vi "allStatus.vi"(4 "intake":bool, 6 "drive":bool, 8 "gear":bool, 9 "shooter":bool, 10 "hopper1":bool, 11 "hopper0":bool) -> ()   [LabVIEW 2016]
uses:
  2ndContollerStatus.vi
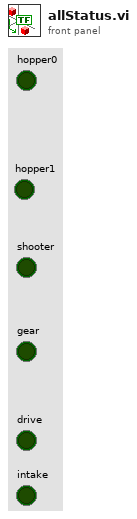
[diagram p1: front panel]
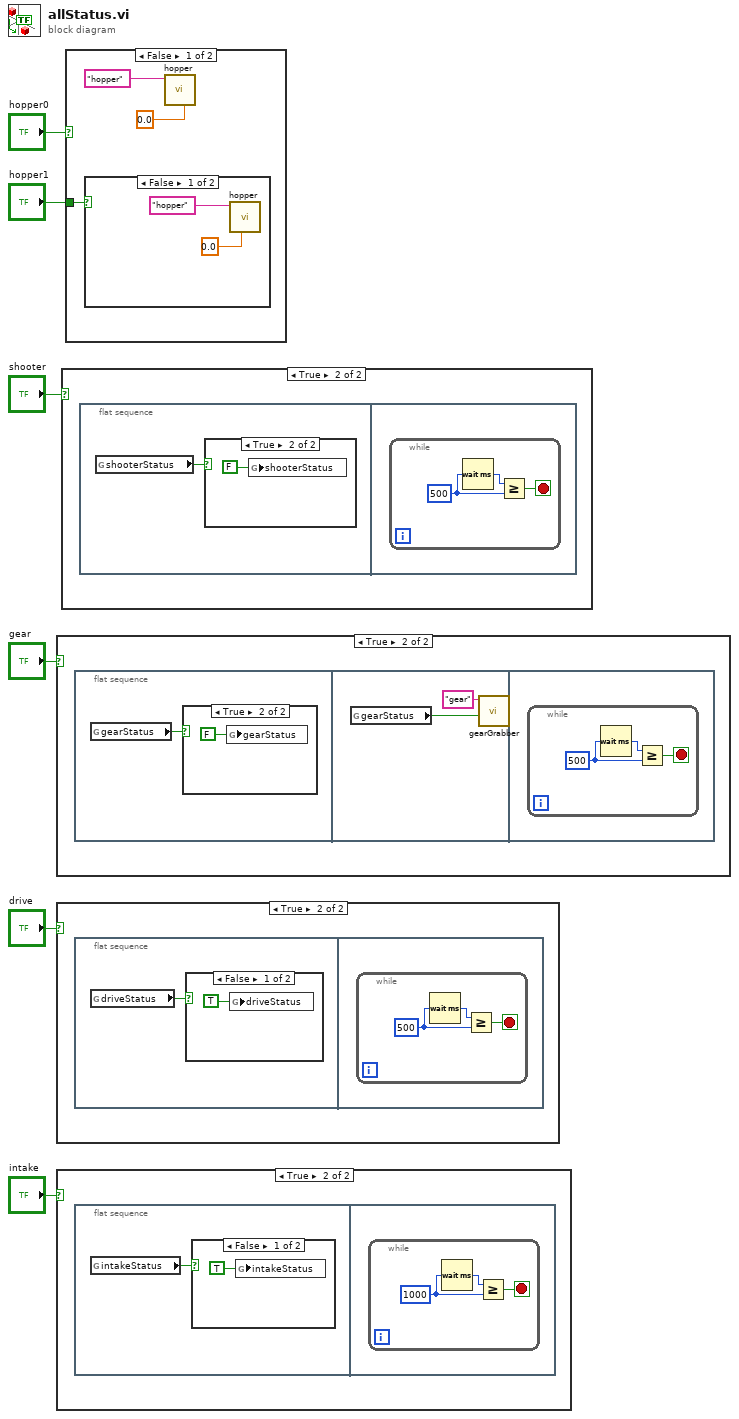
[diagram p0: block diagram]
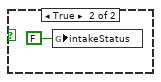
[diagram p3: hidden frame]
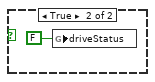
[diagram p5: hidden frame]
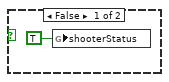
[diagram p7: hidden frame]
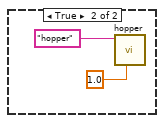
[diagram p8: hidden frame]
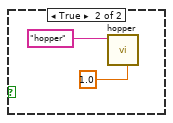
[diagram p9: hidden frame]
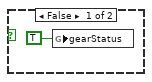
[diagram p11: hidden frame]
diagram:
  n1 = case shown="True" "gear" {
    frame False {
    }
    frame True {
      n2 = flat-sequence {
        frame #0 {
          n3 = global read "2ndContollerStatus.vi" "gearStatus"() -> (w7:bool)
          n4 = case shown="True" w7 {
            frame False {
              n5 = global write "2ndContollerStatus.vi" "gearStatus"(TRUE ("gearStatus")) -> ()
            }
            frame True {
              n6 = global write "2ndContollerStatus.vi" "gearStatus"(FALSE ("gearStatus")) -> ()
            }
          }
        }
        frame #1 {
          n7 = global read "2ndContollerStatus.vi" "gearStatus"() -> (w10:bool)
          n8 = call "gearGrabber.vi"("gearStatus"=w10, "gear"="gear") -> ()  [unwired: 9 in, 1 out]
        }
        frame #2 {
          n9 = while {
            stop <- w14 stop-if-true
            w12 = u32 500 ("milliseconds to wait")
            n10 = Wait (ms)(milliseconds to wait=w12) -> (millisecond timer value=w13:u32)
            n11 = Greater Or Equal?(x=w13, y=w12) -> (x >= y?=w14:bool)
          }
        }
      }
    }
  }
  n12 = case shown="True" "drive" {
    frame False {
    }
    frame True {
      n13 = flat-sequence {
        frame #0 {
          n14 = global read "2ndContollerStatus.vi" "driveStatus"() -> (w15:bool)
          n15 = case shown="False" w15 {
            frame False {
              n16 = global write "2ndContollerStatus.vi" "driveStatus"(TRUE ("driveStatus")) -> ()
            }
            frame True {
              n17 = global write "2ndContollerStatus.vi" "driveStatus"(FALSE ("driveStatus")) -> ()
            }
          }
        }
        frame #1 {
          n18 = while {
            stop <- w18 stop-if-true
            w20 = u32 500 ("milliseconds to wait")
            n19 = Wait (ms)(milliseconds to wait=w20) -> (millisecond timer value=w19:u32)
            n20 = Greater Or Equal?(x=w19, y=w20) -> (x >= y?=w18:bool)
          }
        }
      }
    }
  }
  n21 = case shown="True" "intake" {
    frame False {
    }
    frame True {
      n22 = flat-sequence {
        frame #0 {
          n23 = global read "2ndContollerStatus.vi" "intakeStatus"() -> (w21:bool)
          n24 = case shown="False" w21 {
            frame False {
              n25 = global write "2ndContollerStatus.vi" "intakeStatus"(TRUE ("intakeStatus")) -> ()
            }
            frame True {
              n26 = global write "2ndContollerStatus.vi" "intakeStatus"(FALSE ("intakeStatus")) -> ()
            }
          }
        }
        frame #1 {
          n27 = while {
            stop <- w24 stop-if-true
            w26 = u32 1000 ("milliseconds to wait")
            n28 = Wait (ms)(milliseconds to wait=w26) -> (millisecond timer value=w25:u32)
            n29 = Greater Or Equal?(x=w25, y=w26) -> (x >= y?=w24:bool)
          }
        }
      }
    }
  }
  n30 = case shown="True" "shooter" {
    frame False {
    }
    frame True {
      n31 = flat-sequence {
        frame #0 {
          n32 = global read "2ndContollerStatus.vi" "shooterStatus"() -> (w27:bool)
          n33 = case shown="True" w27 {
            frame False {
              n34 = global write "2ndContollerStatus.vi" "shooterStatus"(TRUE ("shooterStatus")) -> ()
            }
            frame True {
              n35 = global write "2ndContollerStatus.vi" "shooterStatus"(FALSE ("shooterStatus")) -> ()
            }
          }
        }
        frame #1 {
          n36 = while {
            stop <- w30 stop-if-true
            w32 = u32 500 ("milliseconds to wait")
            n37 = Wait (ms)(milliseconds to wait=w32) -> (millisecond timer value=w31:u32)
            n38 = Greater Or Equal?(x=w31, y=w32) -> (x >= y?=w30:bool)
          }
        }
      }
    }
  }
  n39 = case shown="False" "hopper0" {
    tunnel: "hopper1" -> [w35 _]
    frame False {
      n40 = case shown="False" w35 {
        frame False {
          n41 = call "hopper.vi"("Left axis value"=0.0 ("Right axis value"), "hopper"="hopper") -> ()  [unwired: 9 in, 1 out]
        }
        frame True {
          n42 = call "hopper.vi"("Left axis value"=1.0, "hopper"="hopper") -> ()  [unwired: 9 in, 1 out]
        }
      }
      n43 = call "hopper.vi"("Right axis value"=0.0, "hopper"="hopper") -> ()  [unwired: 9 in, 1 out]
    }
    frame True {
      n44 = call "hopper.vi"("Right axis value"=1.0, "hopper"="hopper") -> ()  [unwired: 9 in, 1 out]
    }
  }
